vi "Setra Main.vi"(0 "VISA resource name":refnum<visa-resource-name>="SETRA", 1 "Runtime Gather?":bool, 11 "Error In":errorcluster) -> (4 "Weight Output":dbl, 6 "Weight Output (String)":string, 15 "Error Out":errorcluster)   [LabVIEW 2020]
uses:
  Type Definitions/Setra Commands.ctl
panel:
  in  "Tab Control":enum32{"Main", "Configuration"}(tab)
  in  "Accept Reading":bool
  out "Description":string="Setra Scale Reading"
  in  "Weight (lbs)":dbl
  out "Stable Reading":bool
  in  "Read Scale":bool
  in  "Zero":bool
  out "read buffer":string
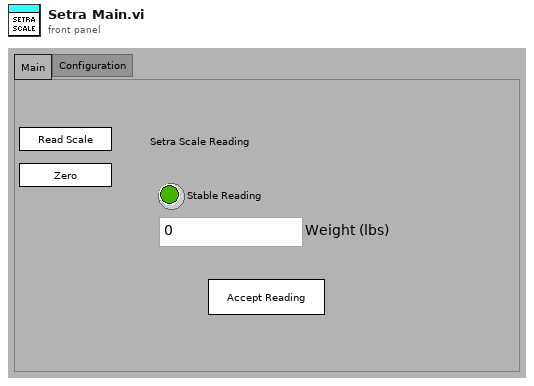
[diagram p1: front panel]
types:
  T1 = typedef "Setra Commands.ctl" = string
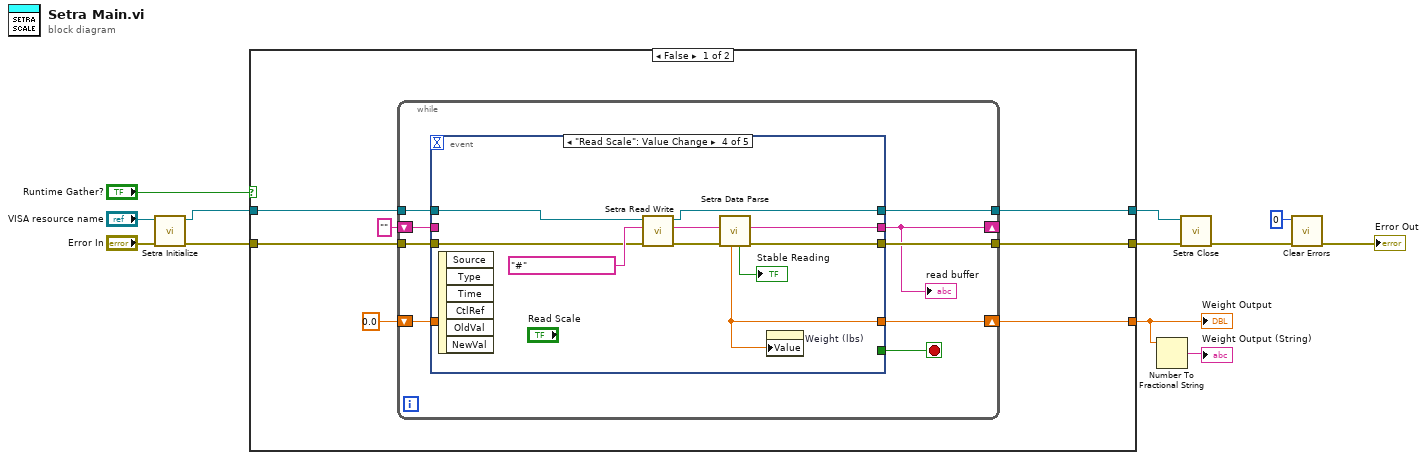
[diagram p0: block diagram]
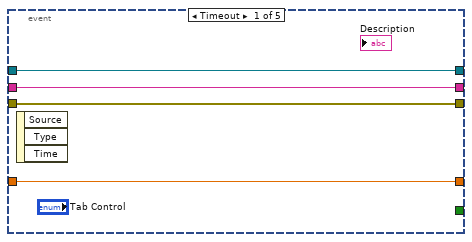
[diagram p2: hidden frame]
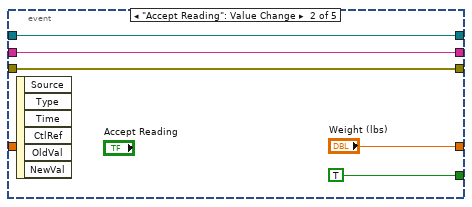
[diagram p3: hidden frame]
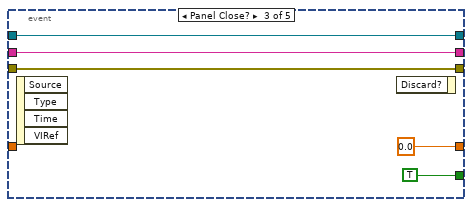
[diagram p4: hidden frame]
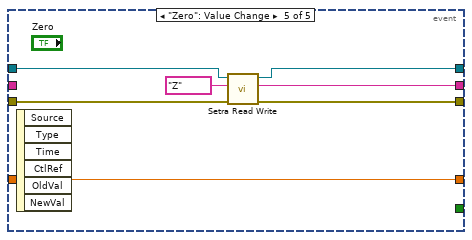
[diagram p5: hidden frame]
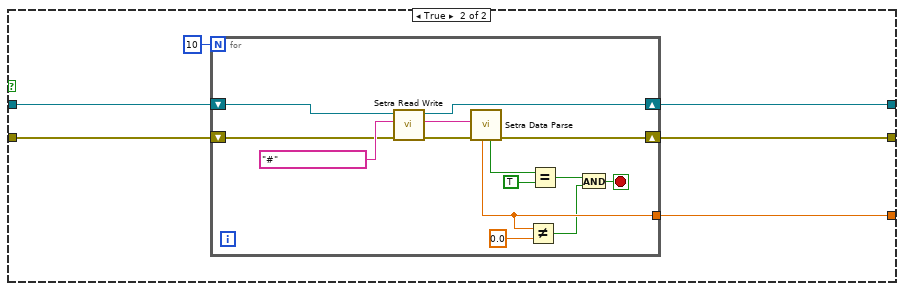
[diagram p6: hidden frame]
diagram:
  n1 = call "Setra Initialize.vi"("Error In"="Error In", "VISA Refnum in"="VISA resource name") -> ("Error Out"=w9:errorcluster, "VISA Refnum out"=w10:refnum<visa-resource-name>)  [unwired: 8 in]
  n2 = case shown="False" "Runtime Gather?" {
    tunnel: w10 -> [w15 w60]
    tunnel: w9 -> [w14 w61]
    tunnel: [w19 w64] -> w8
    tunnel: [w13 w65] -> w7
    tunnel: [w16 w63] -> w3
    frame False {
      n3 = while {
        tunnel: w15 -> [w27]
        tunnel: w14 -> [w28]
        tunnel: [w26] -> w19
        tunnel: [w23] -> w13
        shift-right: [w22] -> _
        shift-left: "" -> [w25]
        shift-right: [w21] -> w16
        shift-left: 0.0 ("Weight") -> [w20]
        stop <- w24 stop-if-true
        n4 = event shown="[3] \"Read Scale\": Value Change" {
          selector: _ -> [_ _ _ _ _]
          dyn-events: _ -> [_ _ _ _ _]
          timeout: _ -> [_ _ _ _ _]
          tunnel: w28 -> [w32 w35 w41 w50 w58]
          tunnel: w27 -> [w31 w34 w40 w51 w57]
          tunnel: [w30 w37 w42 w43 w56] -> w22
          tunnel: [w32 w35 w41 w47 w55] -> w23
          tunnel: [w31 w34 w40 w49 w54] -> w26
          tunnel: w25 -> [w30 w37 w42 _ _]
          tunnel: [_ TRUE ("Accept Reading") TRUE ("Accept Reading") _ _] -> w24
          tunnel: [w29 "Weight (lbs)" 0.0 ("Weight") w45 w53] -> w21
          tunnel: w20 -> [w29 _ _ _ w53]
          event Timeout {
            n5 = event-data() -> ()  [unwired: 1 in, 3 out]
          }
          event "Accept Reading": Value Change {
            n6 = event-data() -> ()  [unwired: 1 in, 6 out]
          }
          event Panel Close? {
            n7 = event-data() -> ()  [unwired: 1 in, 4 out]
            n8 = event-data() -> ()  [unwired: 2 in, 1 out]
          }
          event "Read Scale": Value Change {
            n9 = event-data() -> ()  [unwired: 1 in, 6 out]
            n10 = call "Setra Read Write.vi"("Error In"=w50, "Setra Command"=T1 "#", "VISA (Input)"=w51) -> ("Error Out"=w48:errorcluster, "read buffer"=w44:string, "VISA Refnum (Output)"=w49:refnum<visa-resource-name>)  [unwired: 6 in]
            n11 = call "Setra Data Parse.vi"("Error In"=w48, "Input Data"=w44) -> ("Error Out"=w47:errorcluster, "Output Data"=w43:string, "Data & Stability"=→"Stable Reading":bool, "Weight"=w45:dbl)  [unwired: 6 in]
            n12 = property on="Weight (lbs)" class="DigNum (strict)"("Value"=w45) -> ()  [unwired: 2 in, 2 out]
          }
          event "Zero": Value Change {
            n13 = event-data() -> ()  [unwired: 1 in, 6 out]
            n14 = call "Setra Read Write.vi"("Error In"=w58, "Setra Command"=T1 "Z" ("write buffer"), "VISA (Input)"=w57) -> ("Error Out"=w55:errorcluster, "read buffer"=w56:string, "VISA Refnum (Output)"=w54:refnum<visa-resource-name>)  [unwired: 6 in]
          }
        }
        "read buffer" <- w22
      }
    }
    frame True {
      n15 = for {
        N: 10 -> [_]
        tunnel: [w69] -> w63
        shift-right: [w75] -> w65
        shift-left: w61 -> [w76]
        shift-right: [w74] -> w64
        shift-left: w60 -> [w73]
        stop <- w66 stop-if-true
        n16 = call "Setra Read Write.vi"("Error In"=w76, "Setra Command"=T1 "#", "VISA (Input)"=w73) -> ("Error Out"=w78:errorcluster, "read buffer"=w77:string, "VISA Refnum (Output)"=w74:refnum<visa-resource-name>)  [unwired: 6 in]
        n17 = call "Setra Data Parse.vi"("Error In"=w78, "Input Data"=w77) -> ("Error Out"=w75:errorcluster, "Data & Stability"=w72:bool, "Weight"=w69:dbl)  [unwired: 6 in, 1 out]
        n18 = Not Equal?(x=w69, y=0.0) -> (x != y?=w67:bool)
        n19 = Equal?(x=w72, y=TRUE) -> (x = y?=w70:bool)
        n20 = And(x=w70, y=w67) -> (x .and. y?=w66:bool)
      }
    }
  }
  "Weight Output" <- w3
  n21 = Number To Fractional String(number=w3) -> (F-format string=→"Weight Output (String)":string)  [unwired: 3 in]
  n22 = call "Setra Close.vi"("Error In"=w7, "VISA Refnum in"=w8) -> ("Error Out"=w6:errorcluster)  [unwired: 9 in]
  n23 = call <vilib>:"Clear Errors.vi"("error in (no error)"=w6, "specific error code to clear (0: all)"=0) -> ("error out"=→"Error Out":errorcluster)  [unwired: 4 in, 1 out]
